vi "Global.vi"() -> ()   [LabVIEW 2011, in "IVI DC Power Supply Custom Device.lvlib"]
uses:
  IVI DC Power Supply Custom Device.lvlib
panel:
  in  "Desired Loop Rate":string="Desired Loop Rate"
  in  "Limit Behaviour":string="Limit Behaviour"
  in  "Channel settings GUID":string="15DB30E4-6DFE-7F16-D974-C1D3A3D1FF8B"
  in  "Chan Protect GUID":string="2F57B30F-F7F9-BC70-992A-D64B2B0468D2"
  in  "Over Current":string="Over Current"
  in  "Over Voltage":string="Over Voltage"
  in  "Actual Voltage":string="Actual Voltage"
  in  "OVP Limit":string="OVP Limit"
  in  "OVP Enabled":string="OVP Enabled"
  in  "Channel Page GUID":string="B9A35958-4FA4-E2BC-5A53-1D7326B1BD9E"
  in  "Channel #":string="Channel #"
  in  "Current Limit":string="Current Limit"
  in  "Output Voltage":string="Output Voltage"
  in  "Logical Name":string="Logical Name"
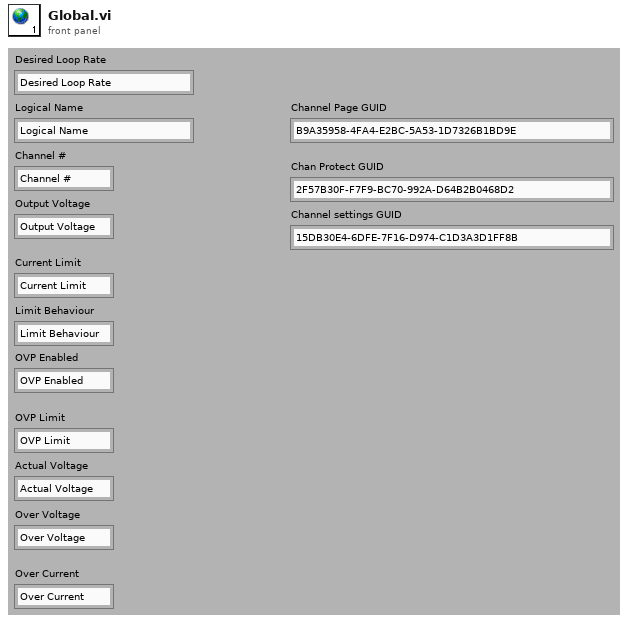
[diagram p1: front panel]
diagram:
